vi "niRFUtil FTW Generate Flat FIR Filter.vi"(1 "Minimum Selectivity (dB)":dbl=70.0 format="%.2f", 2 "Sampling Rate (Hz)":dbl=500000.0 format="%^.3e", 3 "Bandwidth (Hz)":dbl=500000.0 format="%^.3e") -> (0 "Filter":T1 {"y" min=0 max=127 format="%.2f"; "dx" format="%^.2e"; "x0" format="%^.2e"})   [LabVIEW 2015, in "niRFUtil.lvlib"]
doc: "(c) Copyright 2006, National Instruments, Inc. This VI may not be duplicated, sold, or distributed without written consent from National Instruments."
uses:
  niRFUtil.lvlib
  Includes/niRFUtil INC Real Waveform.ctl
  Includes/niRFUtil INC Real Array.ctl
  <vilib>/Analysis/4window.llb/windowTd.ctl
  <vilib>/Analysis/NI_AALBase.lvlib
  <vilib>/Analysis/NI_AALPro.lvlib
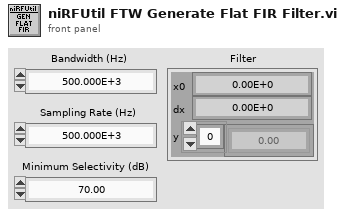
[diagram p1: front panel]
types:
  T1 = typedef "niRFUtil.lvlib/niRFUtil INC Real Waveform.ctl" = cluster{"x0":dbl, "dx":dbl, "y":T2}
  T2 = typedef "niRFUtil.lvlib/niRFUtil INC Real Array.ctl" = sgl[]
  T3 = enum32{"Lowpass", "Highpass", "Bandpass", "Bandstop"}
  T4 = cluster{"Sampling Rate (Hz)":dbl, "Bandwidth (Hz)":dbl, "Minimum Selectivity (dB)":dbl}
  T5 = cluster{"Sampling Rate (Hz)":bool, "Bandwidth (Hz)":bool, "Minimum Selectivity (dB)":bool}
  T6 = typedef "NI_AALPro.lvlib/windowTd.ctl" = u32
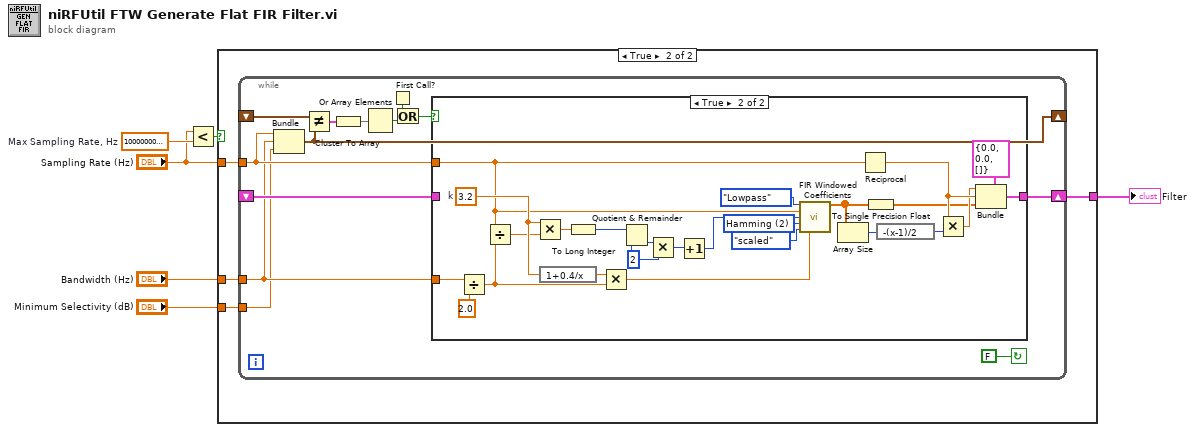
[diagram p0: block diagram]
diagram:
  w3 = 1000000000.0  # Max Sampling Rate, Hz
  n1 = Less?(x="Sampling Rate (Hz)", y=w3) -> (x < y?=w1:bool)
  n2 = case shown="True" w1 {
    tunnel: "Bandwidth (Hz)" -> [_ w10]
    tunnel: "Sampling Rate (Hz)" -> [_ w9]
    tunnel: [_ w8] -> w5
    tunnel: "Minimum Selectivity (dB)" -> [_ w7]
    frame False {
    }
    frame True {
      n3 = while {
        shift-right: [w22] -> w8
        shift-left: _ -> [w21]
        tunnel: w9 -> [w14]
        tunnel: w10 -> [w12]
        shift-right: [w13] -> _
        shift-left: _ -> [w20]
        tunnel: w7 -> [w11]
        stop <- FALSE continue-if-true
        n4 = Bundle("Sampling Rate (Hz)"=w14, "Bandwidth (Hz)"=w12, "Minimum Selectivity (dB)"=w11) -> (w13:T4)  [unwired: 1 out]
        n5 = Not Equal?(x=w20, y=w13) -> (x != y?=w15:T5)
        n6 = Cluster To Array(cluster=w15) -> (array=w19:bool[])
        n7 = Or Array Elements(Boolean array=w19) -> (logical OR=w18:bool)
        n8 = First Call?() -> (First Call?: T/F=w17:bool)
        n9 = Or(x=w17, y=w18) -> (x .or. y?=w16:bool)
        n10 = case shown="True" w16 {
          tunnel: [w24 w36] -> w22
          tunnel: w21 -> [w24 _]
          tunnel: w14 -> [_ w37]
          tunnel: w12 -> [_ w48]
          frame False {
          }
          frame True {
            w33 = 2 ("y")
            w40 = T6 2 items=["Rectangle"=0, "Hanning"=1, "Hamming"=2, "Blackman-Harris"=3, "Exact Blackman"=4, "Blackman"=5, "Flat Top"=6, "4 Term B-Harris "=7, "7 Term B-Harris"=8, "Low Sidelobe"=9, "Blackman Nuttall"=11, "Triangle"=30, "Bartlett-Hanning"=31, "Bohman"=32, "Parzen"=33, "Welch"=34, "Kaiser"=60, "Dolph-Chebyshev"=61, "Gaussian"=62] ("window")
            w43 = 3.2  # k
            n11 = Divide(x=w48, y=2.0) -> (x/y=w38:dbl)
            n12 = Divide(x=w37, y=w38) -> (x/y=w42:dbl)
            n13 = Multiply(x=w43, y=w42) -> (x*y=w44:dbl)
            n14 = expression code="1+0.4/x"(w43) -> (w45:dbl)
            n15 = To Long Integer(number=w44) -> (32bit integer=w35:i32)
            n16 = Multiply(x=w45, y=w38) -> (x*y=w46:dbl)
            n17 = Quotient & Remainder(x=w35, y=w33) -> (floor(x/y)=w34:i32)  [unwired: 1 out]
            n18 = Multiply(x=w34, y=w33) -> (x*y=w32:i32)
            n19 = Increment(x=w32) -> (x+1=w31:i32)
            n20 = call <vilib>:"FIR Windowed Coefficients.vi"("filter type"=T3."Lowpass", "sampling freq: fs"=w37, "taps"=w31, "window"=w40, "option"=enum32{"not scaled", "scaled"}."scaled", "low cutoff freq: fl"=w46) -> ("FIR Windowed Coefficients"=w30:dbl[])  [unwired: 2 in, 7 out]
            n21 = Array Size(array=w30) -> (size(s)=w47:i32)
            n22 = Reciprocal(x=w37) -> (1/x=w28:dbl)
            n23 = To Single Precision Float(number=w30) -> (single precision float=w25:sgl[])
            n24 = expression code="-(x-1)/2"(w47) -> (w29:i32)
            n25 = Multiply(x=w28, y=w29) -> (x*y=w27:dbl)
            n26 = Bundle(cluster=T1 {"x0"=0.0, "dx"=0.0, "y"=[]} ("Filter"), "x0"=w27, "dx"=w28, "y"=w25) -> (w36:T1)
          }
        }
      }
    }
  }
  "Filter" <- w5
